vi "teste_com_RGB.vi"() -> ()   [LabVIEW 2016]
uses:
  parametros.ctl
  <vilib>/NXT/Block Support/NXT_InputPort.ctl
  <vilib>/NXT/Dual Mode Library/Display/clearDisplay.vi
  <vilib>/NXT/Dual Mode Library/Display/drawText_Center.vi
panel:
  in  "Parâmetros Ini":T1={"Gyro Port"=0, "Sensor - Left"=3, "Sensor - Right"=2, "     Color \nSensor Port"=1, "Kp Front"=0.5, "Motor speed"=-15, "Distance to street"=0.0, "Motor speed turns"=16, "Kp Curvas"=0.0} {"Kp Front" format="%.3f"; "Color \nSensor Port" items=["Port 1", "Port 2", "Port 3", "Port 4"]; "Sensor - Right" items=["Port 1", "Port 2", "Port 3", "Port 4"]; "Sensor - Left" items=["Port 1", "Port 2", "Port 3", "Port 4"]; "Gyro Port" items=["Port 1", "Port 2", "Port 3", "Port 4"]}
  out "RGB Color":cluster{"Red":u8, "Green":u8, "Blue":u8}
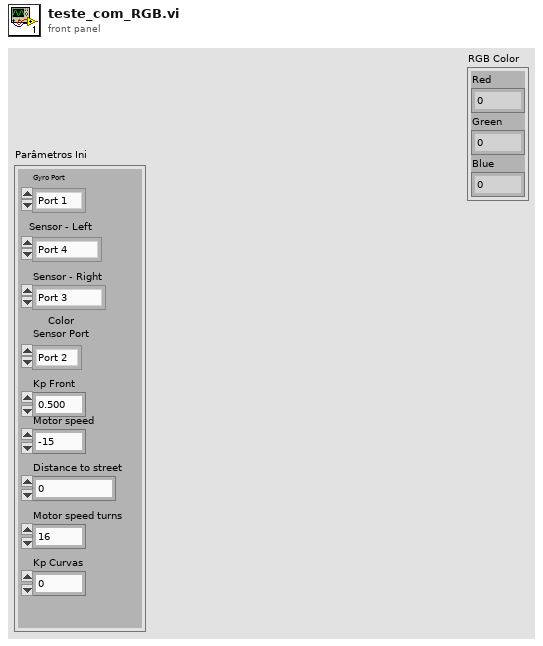
[diagram p1: front panel]
types:
  T1 = typedef "parametros.ctl" = cluster{"Gyro Port":T2, "Sensor - Left":T2, "Sensor - Right":T2, "     Color \nSensor Port":T2, "Kp Front":dbl, "Motor speed":i32, "Distance to street":dbl, "Motor speed turns":i32, "Kp Curvas":dbl}
  T2 = typedef "NXT_InputPort.ctl" = u32
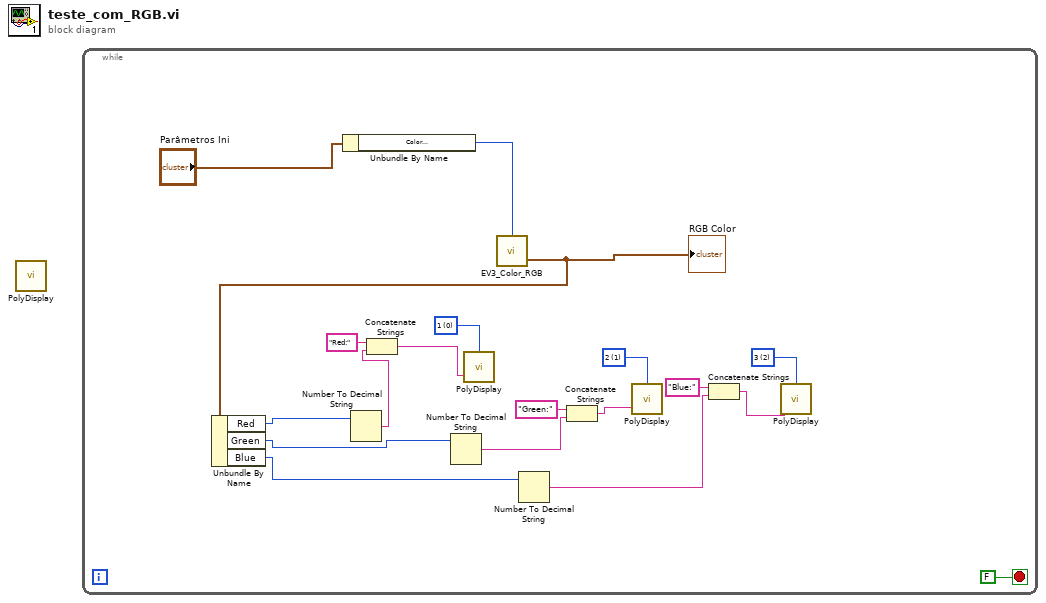
[diagram p0: block diagram]
diagram:
  n1 = call-poly <vilib>:"PolyDisplay.vi"() -> ()  [unwired: 4 in, 1 out]
  n2 = while {
    stop <- FALSE stop-if-true
    w15 = i16 2 items=["1", "2", "3", "4", "5", "6", "7", "8", "9", "10", "11", "12"] ("Line")
    w16 = i16 1 items=["1", "2", "3", "4", "5", "6", "7", "8", "9", "10", "11", "12"] ("Line")
    w17 = i16 0 items=["1", "2", "3", "4", "5", "6", "7", "8", "9", "10", "11", "12"] ("Line")
    n3 = Unbundle By Name("Parâmetros Ini") -> ("Color \nSensor Port"=w18:T2)
    n4 = call <vilib>:"EV3_Color_RGB.vi"("Port (Port 1)"=w18) -> ("RGB Color"=w14:cluster{"Red":u8, "Green":u8, "Blue":u8})  [unwired: 2 in, 1 out]
    "RGB Color" <- w14
    n5 = Unbundle By Name(w14) -> ("Red"=w13:u8, "Green"=w12:u8, "Blue"=w11:u8)
    n6 = Number To Decimal String(number=w13) -> (decimal integer string=w7:string)  [unwired: 1 in]
    n7 = Concatenate Strings("Red:" ("string"), w7) -> (w6:string)
    n8 = Number To Decimal String(number=w12) -> (decimal integer string=w4:string)  [unwired: 1 in]
    n9 = call-poly <vilib>:"PolyDisplay.vi"("Text"=w6, "Line"=w17) -> ()  [unwired: 2 in, 1 out]
    n10 = Number To Decimal String(number=w11) -> (decimal integer string=w2:string)  [unwired: 1 in]
    n11 = Concatenate Strings("Green:" ("string"), w4) -> (w5:string)
    n12 = call-poly <vilib>:"PolyDisplay.vi"("Text"=w5, "Line"=w16) -> ()  [unwired: 2 in, 1 out]
    n13 = Concatenate Strings("Blue:" ("string"), w2) -> (w3:string)
    n14 = call-poly <vilib>:"PolyDisplay.vi"("Text"=w3, "Line"=w15) -> ()  [unwired: 2 in, 1 out]
  }
